vi "mainer.vi"() -> ()   [LabVIEW 2017]
uses:
  mark_10_setting_1.ctl
  acquire_enum.ctl
  serial_setting_1.ctl
  <vilib>/DAQmx/read.llb/DAQmx Read (Analog 1D Wfm NChan NSamp).vi
  <vilib>/DAQmx/miscellaneous.llb/DAQmx Fill In Error Info.vi
  <vilib>/Instr/_visa.llb/VISA Configure Serial Port (Instr).vi
panel:
  in  "Trigger Force(N)":dbl
  in  "Stop Trigger":bool
  in  "Move":bool
  in  "Target Distance":dbl
  in  "Sampling Rate(Hz)":dbl
  out "dt(ms)":u32
  in  "Reset Cycle":bool
  out "Readings":cluster{dbl, "Numeric":dbl, "Numeric":dbl}(graph)
  in  "Record":bool
  in  "Log TXT file":path
  out "Cycles":string
  in  "Zero":bool
  in  "Stop Button":bool
  out "Current Status":string
  in  "Auto Zero":bool
  out "Travel":string
  out "Load":string
  in  "Mark-10":refnum<visa-resource-name>
  in  "Down Button":bool
  in  "Up Button":bool
  in  "Exit":bool
  in  "Mark-10 Setup":bool
  # "Max 45Hz!"
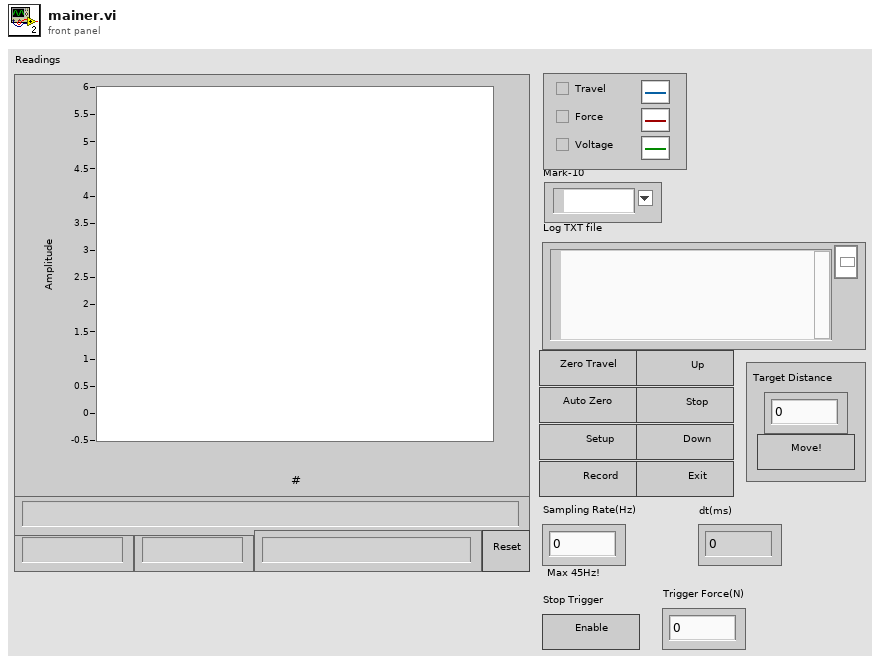
[diagram p1: front panel]
types:
  T1 = typedef "acquire_enum.ctl" = enum16{"Move to Target", "Connect to NIDAQ", "Connect to Mark-10", "Reset Cycle", "Open Mark-10 Setup", "Auto Zero", "Zero", "Stop", "Down", "Up", "Initialize", "Exit", "New Log Path", "Acquire"}
  T2 = typedef "mark_10_setting_1.ctl" = cluster{"Speed (mm/min)":dbl, "Up Limit(mm)":dbl, "Down Limit(mm)":dbl, "Cycle Mode":bool, "Number of Cycles":i32, "IsConfigured":bool}
  T3 = cluster{"Move":refnum<vi>, "Mark-10":refnum<vi>, "Mark-10 Setup":refnum<vi>, "Reset Cycle":refnum<vi>, "Stop Button":refnum<vi>, "Log TXT file":refnum<vi>, "Up Button":refnum<vi>, "Down Button":refnum<vi>, "Auto Zero":refnum<vi>, "Zero":refnum<vi>, "Exit":refnum<vi>, "Record":refnum<vi>, "Sampling Rate(Hz)":refnum<vi>}
  T4 = enum8{"Enabled", "Disabled", "Disabled and Grayed Out"}
  T5 = typedef "serial_setting_1.ctl" = cluster{"baud rate":u32, "data bits":u16, "parity":enum16{"None", "Odd", "Even", "Mark", "Space"}, "stop bits":u16, "flow control":u16, "IsConfigured":bool}
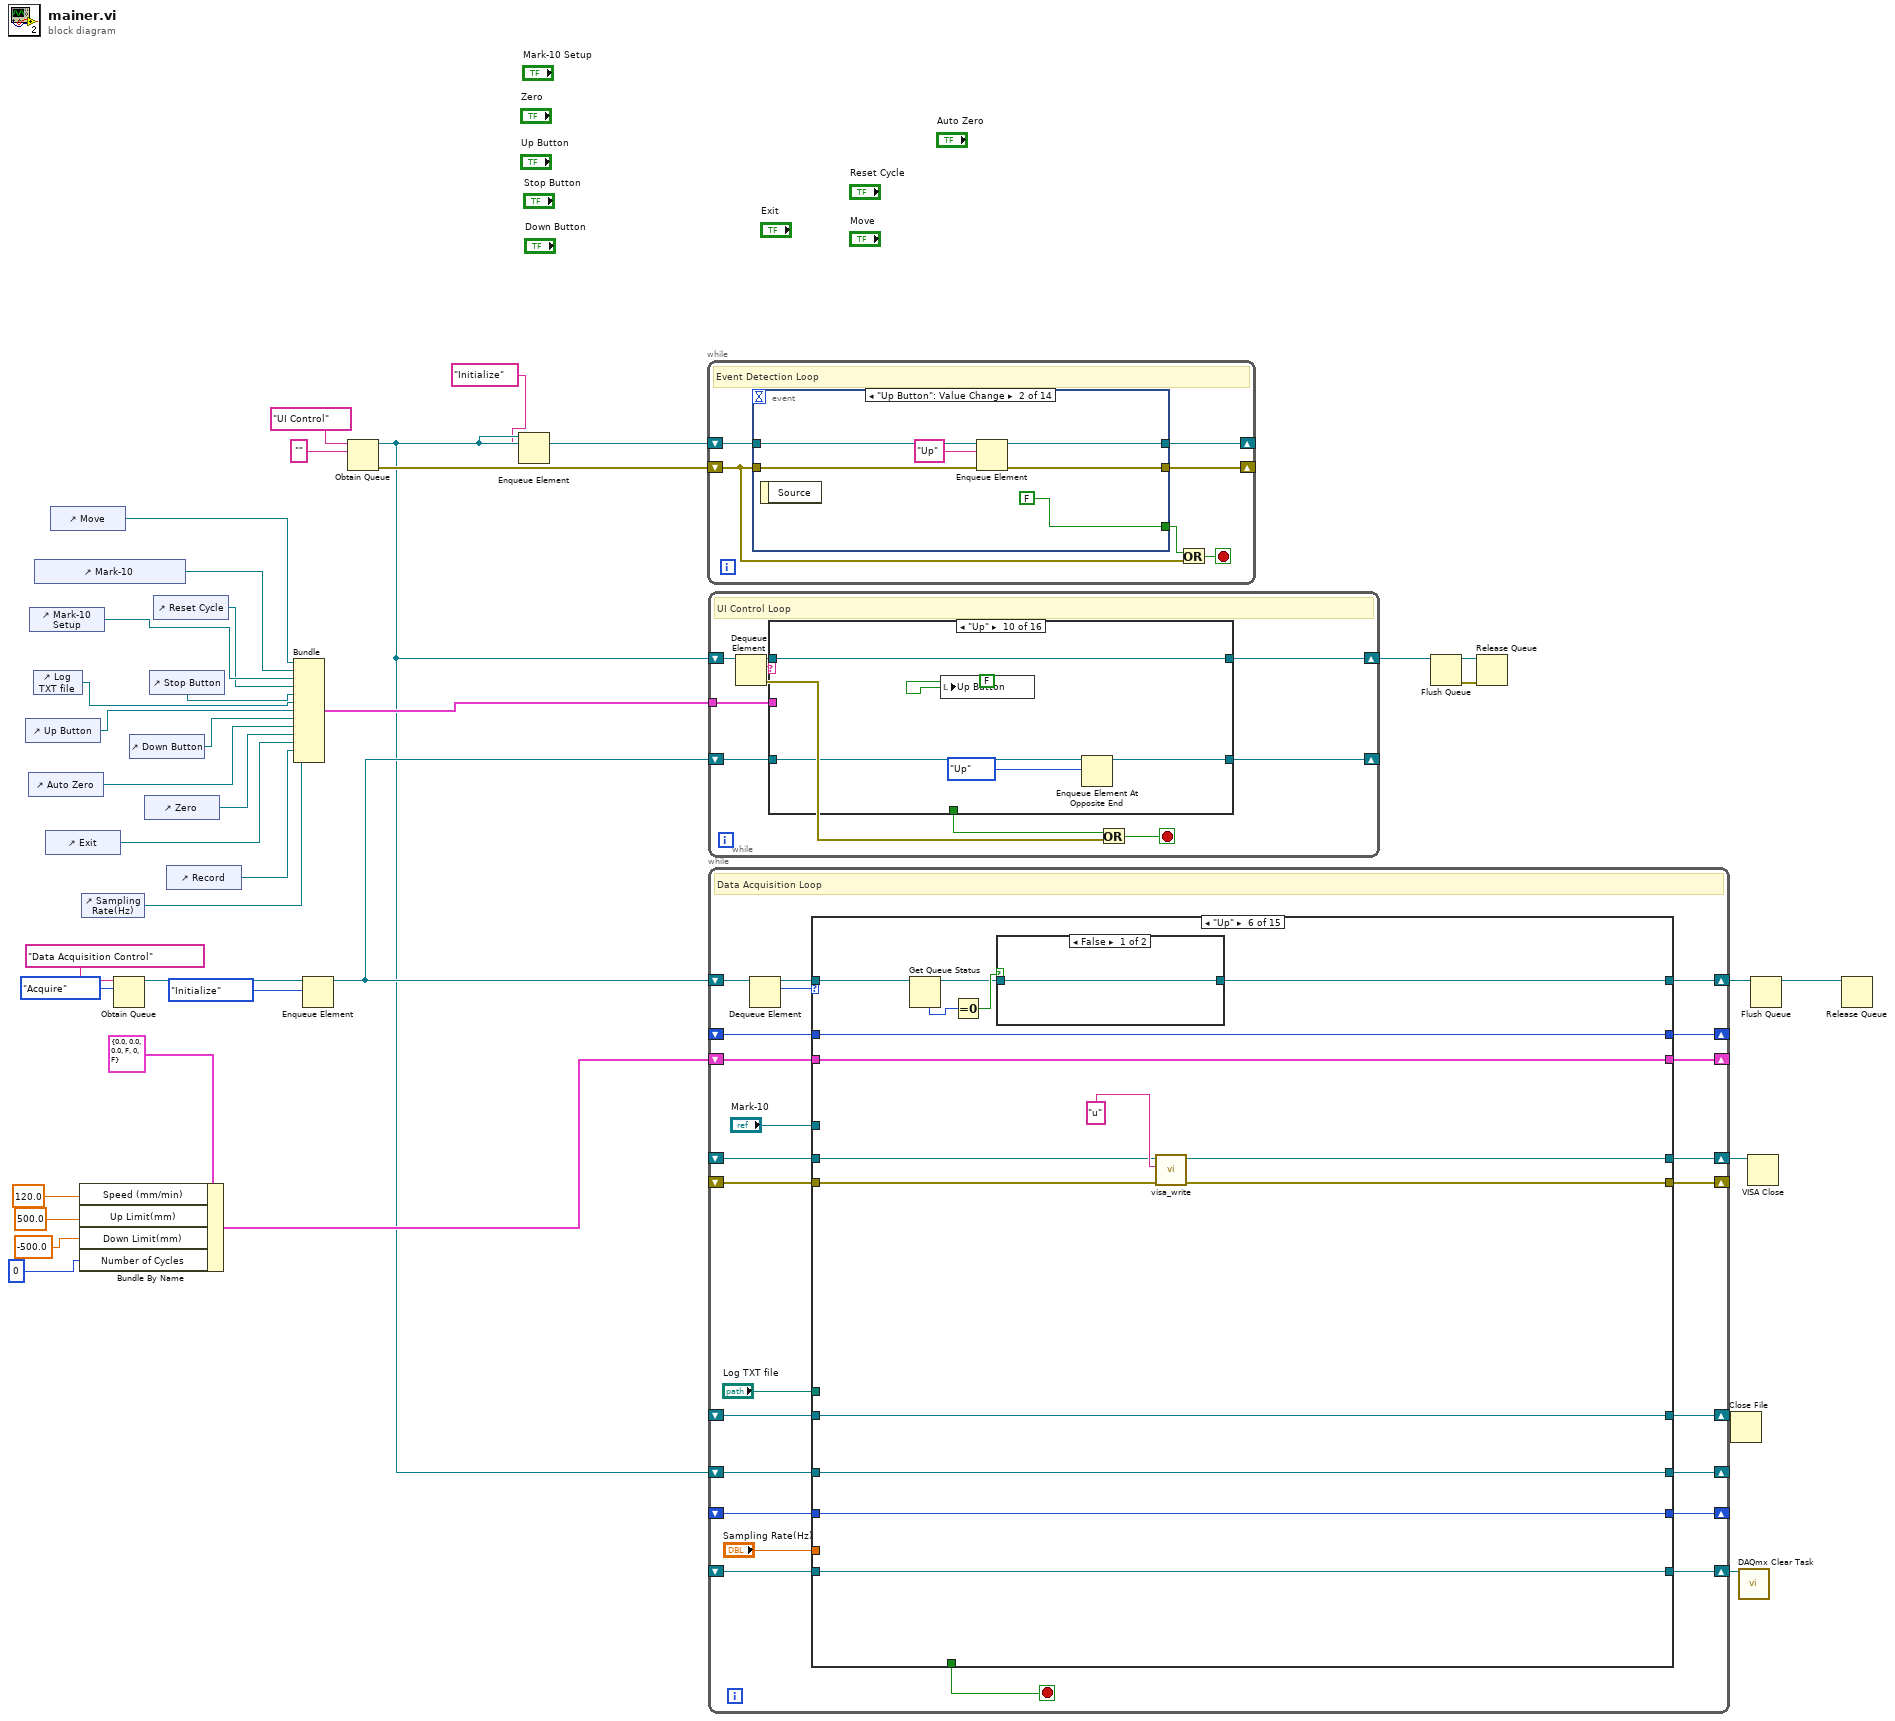
[diagram p0: block diagram]
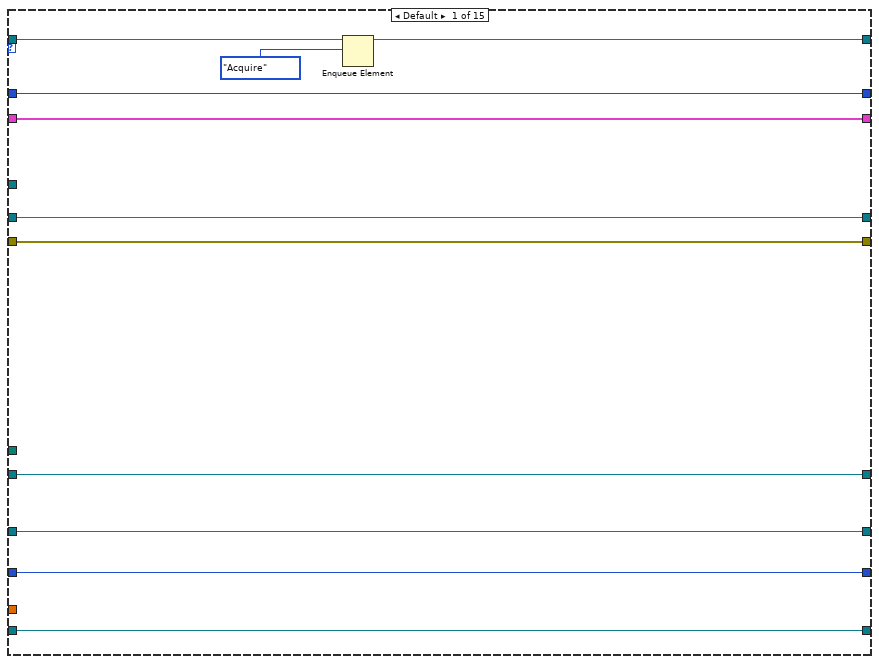
[diagram p2: hidden frame]
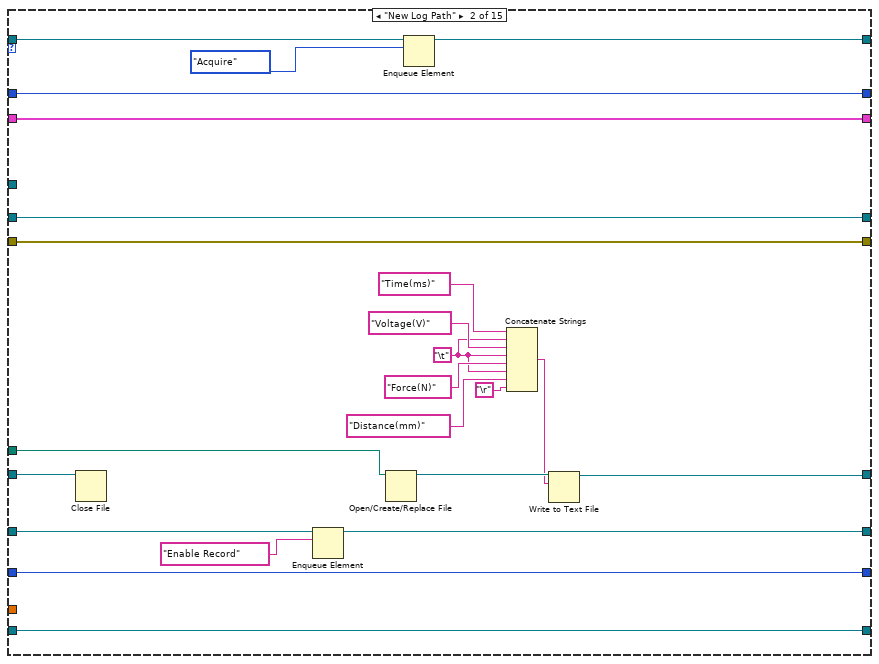
[diagram p3: hidden frame]
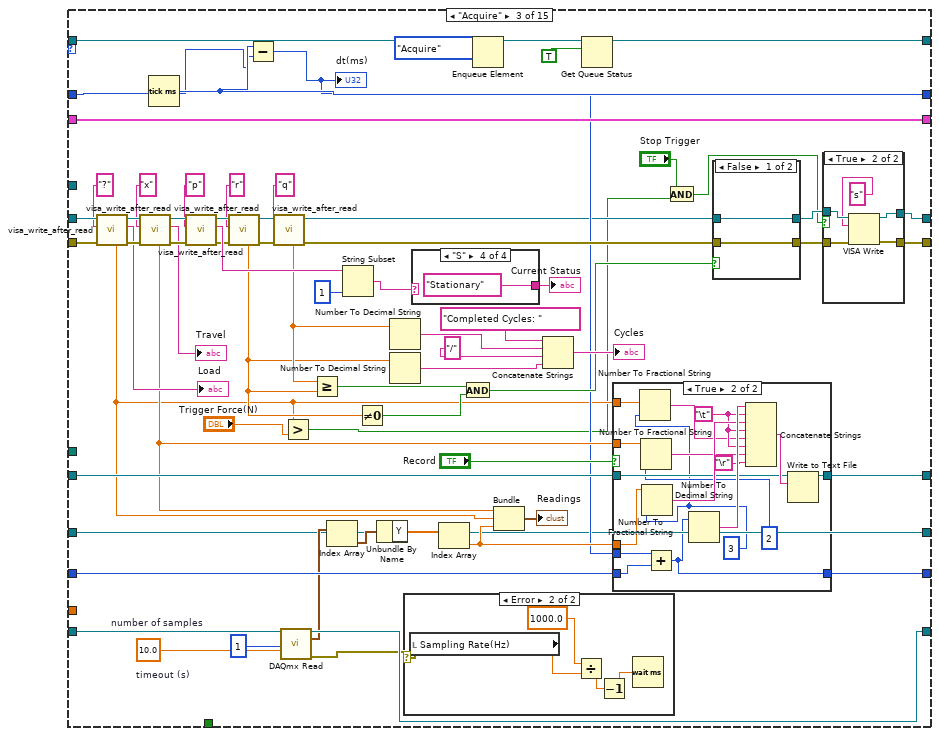
[diagram p4: hidden frame]
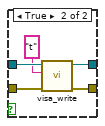
[diagram p7: hidden frame]
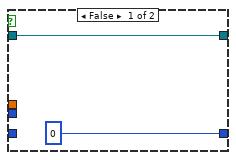
[diagram p8: hidden frame]
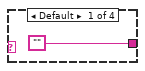
[diagram p9: hidden frame]
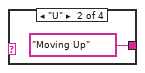
[diagram p10: hidden frame]
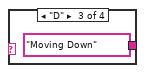
[diagram p11: hidden frame]
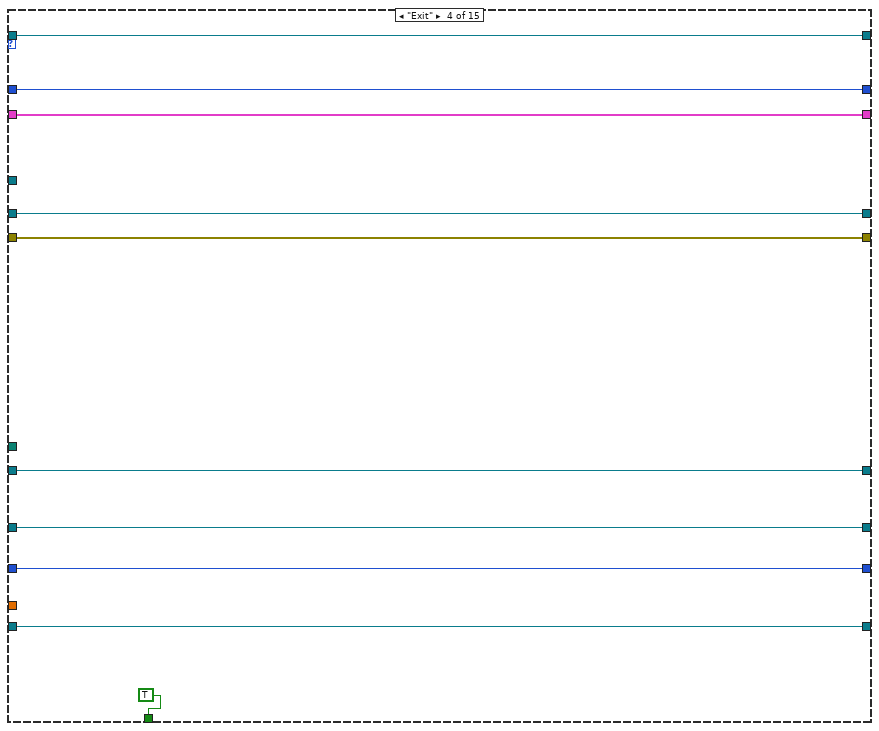
[diagram p12: hidden frame]
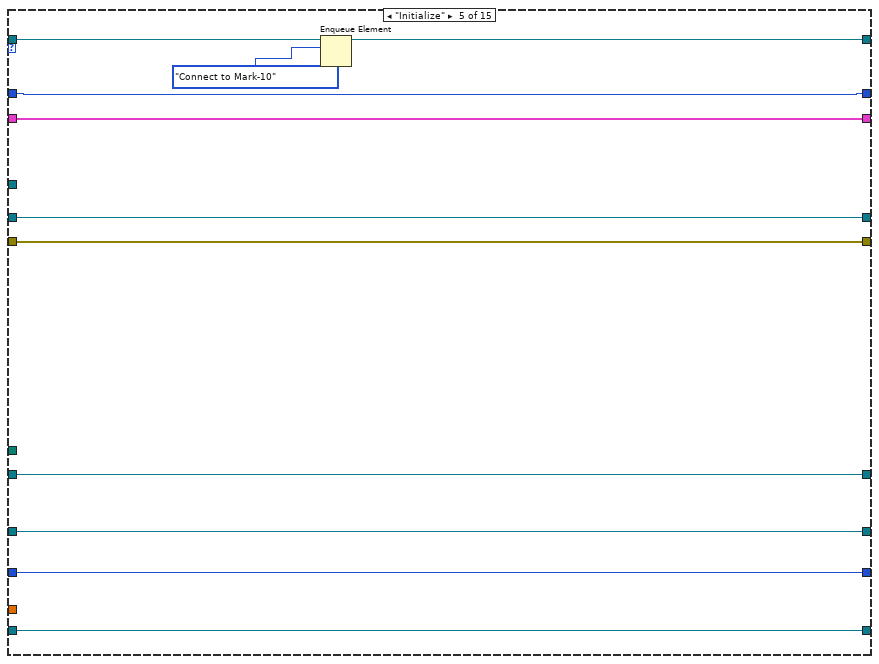
[diagram p13: hidden frame]
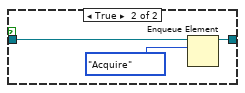
[diagram p14: hidden frame]
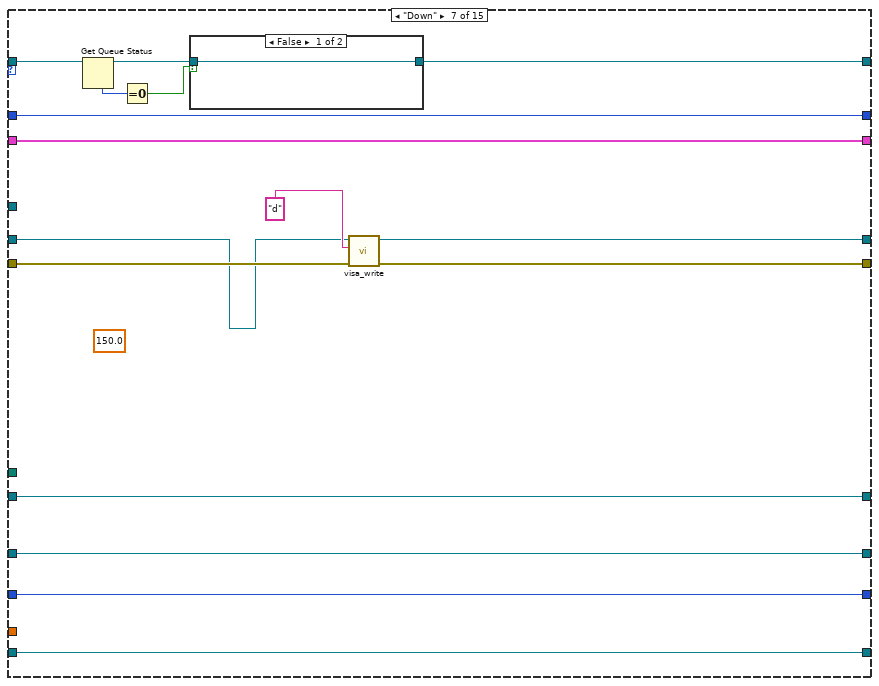
[diagram p15: hidden frame]
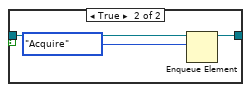
[diagram p16: hidden frame]
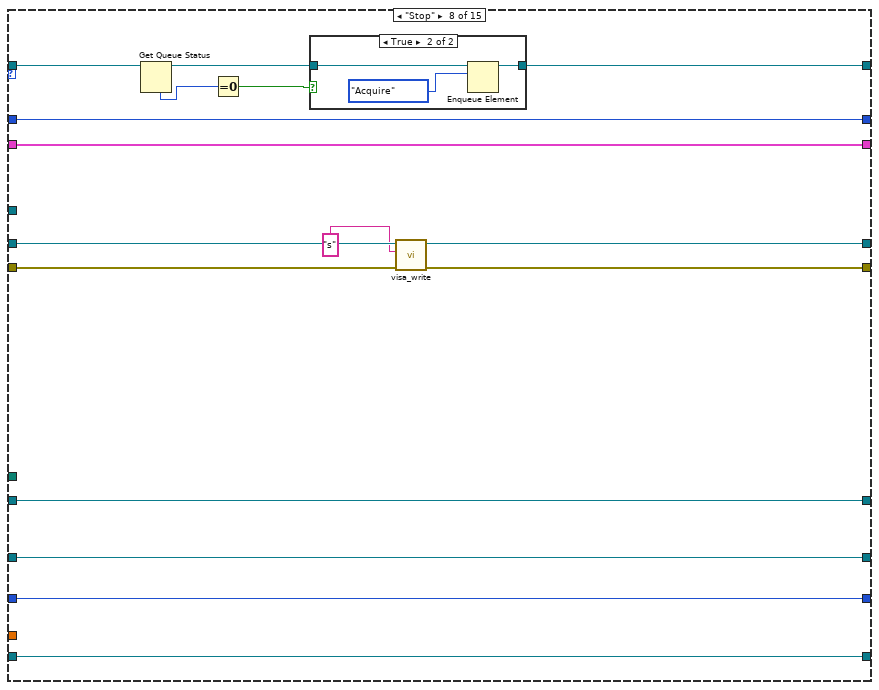
[diagram p17: hidden frame]
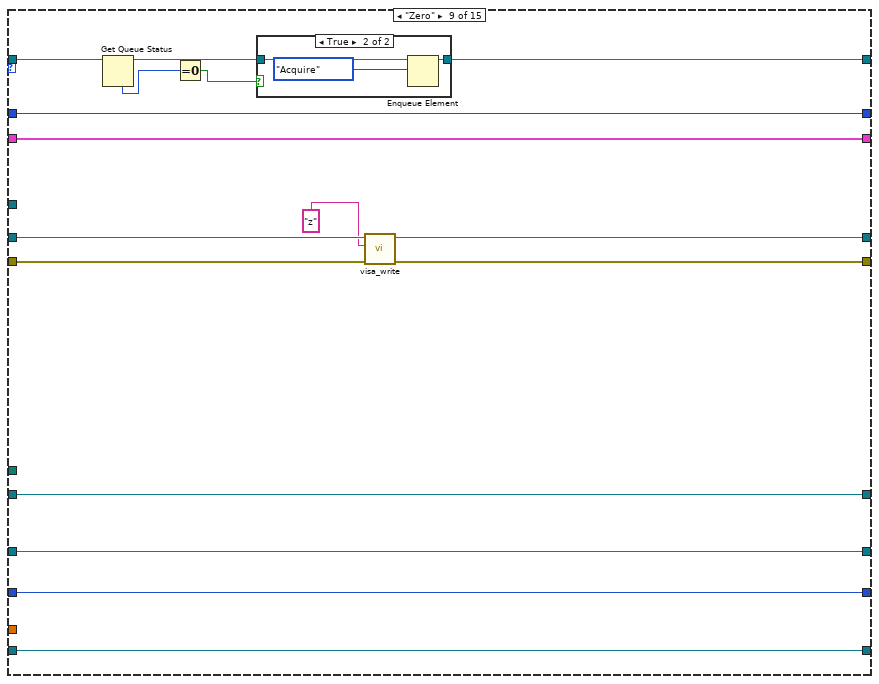
[diagram p19: hidden frame]
diagram:
  n1 = control-ref of="Up Button"() -> (w9:refnum<vi>)
  n2 = control-ref of="Auto Zero"() -> (w7:refnum<vi>)
  n3 = control-ref of="Mark-10 Setup"() -> (w13:refnum<vi>)
  n4 = control-ref of="Log TXT file"() -> (w10:refnum<vi>)
  n5 = control-ref of="Mark-10"() -> (w14:refnum<vi>)
  n6 = control-ref of="Exit"() -> (w5:refnum<vi>)
  n7 = control-ref of="Move"() -> (w15:refnum<vi>)
  n8 = Bundle By Name(cluster=T2 {"Speed (mm/min)"=0.0, "Up Limit(mm)"=0.0, "Down Limit(mm)"=0.0, "Cycle Mode"=FALSE, "Number of Cycles"=0, "IsConfigured"=FALSE} ("Mark-10 Settings"), "Speed (mm/min)"=120.0, "Up Limit(mm)"=500.0, "Down Limit(mm)"=-500.0, "Number of Cycles"=0) -> (w18:T2)
  n9 = control-ref of="Sampling Rate(Hz)"() -> (w1:refnum<vi>)
  n10 = Obtain Queue(name (unnamed)="Data Acquisition Control", element data type=acquire_enum."Acquire") -> (queue out=w29:refnum<queue>)  [unwired: 3 in, 2 out]
  n11 = control-ref of="Down Button"() -> (w8:refnum<vi>)
  n12 = control-ref of="Zero"() -> (w6:refnum<vi>)
  n13 = control-ref of="Stop Button"() -> (w11:refnum<vi>)
  n14 = control-ref of="Reset Cycle"() -> (w12:refnum<vi>)
  n15 = control-ref of="Record"() -> (w4:refnum<vi>)
  n16 = Bundle("Move"=w15, "Mark-10"=w14, "Mark-10 Setup"=w13, "Reset Cycle"=w12, "Stop Button"=w11, "Log TXT file"=w10, "Up Button"=w9, "Down Button"=w8, "Auto Zero"=w7, "Zero"=w6, "Exit"=w5, "Record"=w4, "Sampling Rate(Hz)"=w1) -> (w16:T3)  [unwired: 1 in]
  n17 = Enqueue Element(queue=w29, element=acquire_enum."Initialize") -> (queue out=w27:refnum<queue>)  [unwired: 2 in, 2 out]
  n18 = Obtain Queue(name (unnamed)="UI Control", element data type="") -> (queue out=w3:refnum<queue>, error out=w35:errorcluster)  [unwired: 3 in, 1 out]
  n19 = Enqueue Element(queue=w3, element="Initialize") -> ()  [unwired: 2 in, 3 out]
  n20 = while {
    shift-right: [w43] -> _
    shift-left: w3 -> [w44]
    shift-right: [w42] -> _
    shift-left: w35 -> [w39]
    stop <- w41 stop-if-true
    # "Event Detection Loop"
    n21 = event shown="[1] \"Up Button\": Value Change" {
      selector: _ -> [_ _ _ _ _ _ _ _ _ _ _ _ _ _]
      dyn-events: _ -> [_ _ _ _ _ _ _ _ _ _ _ _ _ _]
      timeout: _ -> [_ _ _ _ _ _ _ _ _ _ _ _ _ _]
      tunnel: [TRUE FALSE FALSE FALSE _ FALSE FALSE FALSE FALSE FALSE FALSE FALSE FALSE TRUE] -> w40
      tunnel: w44 -> [w47 w53 w59 w65 w70 w76 w82 w88 w94 w99 w105 w111 w117 w120]
      tunnel: [w47 w52 w58 w64 w69 w75 w81 w87 w93 w98 w104 w110 w116 w123] -> w43
      tunnel: w39 -> [w46 w51 w57 w63 w67 w74 w80 w86 w92 w97 w103 w109 w115 w119]
      tunnel: [w46 w50 w56 w62 w68 w73 w79 w85 w91 w96 w102 w108 w114 w122] -> w42
      event Timeout {
        n22 = event-data() -> ()  [unwired: 1 in, 1 out]
      }
      event "Up Button": Value Change {
        n23 = event-data() -> ()  [unwired: 1 in, 1 out]
        n24 = Enqueue Element(queue=w53, element="Up", error in (no error)=w51) -> (queue out=w52:refnum<queue>, error out=w50:errorcluster)  [unwired: 1 in, 1 out]
      }
      event "Reset Cycle": Value Change {
        n25 = event-data() -> ()  [unwired: 1 in, 1 out]
        n26 = Enqueue Element(queue=w59, element="Reset Cycle", error in (no error)=w57) -> (queue out=w58:refnum<queue>, error out=w56:errorcluster)  [unwired: 1 in, 1 out]
      }
      event "Stop Button": Value Change {
        n27 = event-data() -> ()  [unwired: 1 in, 2 out]
        n28 = Enqueue Element(queue=w65, element="Stop", error in (no error)=w63) -> (queue out=w64:refnum<queue>, error out=w62:errorcluster)  [unwired: 1 in, 1 out]
      }
      event "Record": Value Change {
        n29 = event-data() -> ()  [unwired: 1 in, 2 out]
        n30 = Enqueue Element(queue=w70, element="Record", error in (no error)=w67) -> (queue out=w69:refnum<queue>, error out=w68:errorcluster)  [unwired: 1 in, 1 out]
      }
      event "Log TXT file": Value Change {
        n31 = event-data() -> ()  [unwired: 1 in, 2 out]
        n32 = Enqueue Element(queue=w76, element="Change Log Path", error in (no error)=w74) -> (queue out=w75:refnum<queue>, error out=w73:errorcluster)  [unwired: 1 in, 1 out]
      }
      event "Sampling Rate(Hz)": Value Change {
        n33 = event-data() -> ()  [unwired: 1 in, 2 out]
        n34 = Enqueue Element(queue=w82, element="Change Sampling Rate", error in (no error)=w80) -> (queue out=w81:refnum<queue>, error out=w79:errorcluster)  [unwired: 1 in, 1 out]
      }
      event "Move": Value Change {
        n35 = event-data() -> ()  [unwired: 1 in, 2 out]
        n36 = Enqueue Element(queue=w88, element="Move", error in (no error)=w86) -> (queue out=w87:refnum<queue>, error out=w85:errorcluster)  [unwired: 1 in, 1 out]
      }
      event "Zero": Value Change {
        n37 = event-data() -> ()  [unwired: 1 in, 2 out]
        n38 = Enqueue Element(queue=w94, element="Zero", error in (no error)=w92) -> (queue out=w93:refnum<queue>, error out=w91:errorcluster)  [unwired: 1 in, 1 out]
      }
      event "Down Button": Value Change {
        n39 = event-data() -> ()  [unwired: 1 in, 1 out]
        n40 = Enqueue Element(queue=w99, element="Down", error in (no error)=w97) -> (queue out=w98:refnum<queue>, error out=w96:errorcluster)  [unwired: 1 in, 1 out]
      }
      event "Mark-10": Value Change {
        n41 = event-data() -> ()  [unwired: 1 in, 2 out]
        n42 = Enqueue Element(queue=w105, element="Connect to Mark-10", error in (no error)=w103) -> (queue out=w104:refnum<queue>, error out=w102:errorcluster)  [unwired: 1 in, 1 out]
      }
      event "Mark-10 Setup": Value Change {
        n43 = event-data() -> ()  [unwired: 1 in, 2 out]
        n44 = Enqueue Element(queue=w111, element="Open Mark-10 Setup", error in (no error)=w109) -> (queue out=w110:refnum<queue>, error out=w108:errorcluster)  [unwired: 1 in, 1 out]
      }
      event "Auto Zero": Value Change {
        n45 = event-data() -> ()  [unwired: 1 in, 2 out]
        n46 = Enqueue Element(queue=w117, element="Auto Zero", error in (no error)=w115) -> (queue out=w116:refnum<queue>, error out=w114:errorcluster)  [unwired: 1 in, 1 out]
      }
      event "Exit": Value Change {
        n47 = event-data() -> ()  [unwired: 1 in, 1 out]
        n48 = Enqueue Element(queue=w120, element="Exit", error in (no error)=w119) -> (queue out=w123:refnum<queue>, error out=w122:errorcluster)  [unwired: 1 in, 1 out]
      }
    }
    n49 = Or(x=w40, y=w39) -> (x .or. y?=w41:bool)
  }
  n50 = while {
    shift-right: [w131] -> w25
    shift-left: w3 -> [w134]
    shift-right: [w129] -> _
    shift-left: w27 -> [w130]
    tunnel: w16 -> [w125]
    stop <- w128 stop-if-true
    # "UI Control Loop"
    n51 = Dequeue Element(queue=w134) -> (queue out=w132:refnum<queue>, element=w133:string, error out=w126:errorcluster)  [unwired: 2 in, 1 out]
    n52 = case shown="\"Up\"" w133 {
      tunnel: w132 -> [w136 w137 w145 w150 w154 w159 w163 w167 w172 w173 w179 w189 w194 w199 w204 w209]
      tunnel: [w136 w137 w145 w150 w154 w159 w163 w167 w172 w173 w179 w189 w194 w199 w204 w209] -> w131
      tunnel: [_ _ TRUE _ _ _ _ _ _ _ _ _ _ _ _ _] -> w127
      tunnel: w130 -> [w135 w138 w143 w147 w153 w158 w162 w166 w171 w175 w178 w188 w191 w196 w202 w207]
      tunnel: [w135 w138 w142 w146 w152 w156 w160 w164 w169 w174 w178 w188 w190 w195 w201 w206] -> w129
      tunnel: w125 -> [_ _ _ _ _ _ _ _ _ _ _ w187 _ _ _ _]
      frame Default {
      }
      frame "Record" {
        n53 = control-ref of="Log TXT file"() -> (w139:refnum<vi>)
        n54 = call "toggle_enable.vi"("reference"=w139) -> ()  [unwired: 10 in, 1 out]
      }
      frame "Exit" {
        n55 = local write "Exit"(FALSE) -> ()
        n56 = Enqueue Element(queue=w143, element=acquire_enum."Exit") -> (queue out=w142:refnum<queue>)  [unwired: 2 in, 2 out]
      }
      frame "Open Mark-10 Setup" {
        n57 = local write "Mark-10 Setup"(FALSE) -> ()
        n58 = Enqueue Element(queue=w147, element=acquire_enum."Open Mark-10 Setup") -> (queue out=w146:refnum<queue>)  [unwired: 2 in, 2 out]
      }
      frame "Auto Zero" {
        n59 = local write "Auto Zero"(FALSE) -> ()
        n60 = Enqueue Element(queue=w153, element=acquire_enum."Auto Zero") -> (queue out=w152:refnum<queue>)  [unwired: 2 in, 2 out]
      }
      frame "Change Log Path" {
        n61 = Enqueue Element(queue=w158, element=acquire_enum."New Log Path") -> (queue out=w156:refnum<queue>)  [unwired: 2 in, 2 out]
      }
      frame "Connect to Mark-10" {
        n62 = Enqueue Element(queue=w162, element=acquire_enum."Connect to Mark-10") -> (queue out=w160:refnum<queue>)  [unwired: 2 in, 2 out]
      }
      frame "Change Sampling Rate" {
        n63 = Enqueue Element(queue=w166, element=acquire_enum."Connect to NIDAQ") -> (queue out=w164:refnum<queue>)  [unwired: 2 in, 2 out]
      }
      frame "Move" {
        n64 = Enqueue Element(queue=w171, element=acquire_enum."Move to Target") -> (queue out=w169:refnum<queue>)  [unwired: 2 in, 2 out]
        n65 = local write "Move"(FALSE) -> ()
      }
      frame "Up" {
        n66 = local write "Up Button"(FALSE) -> ()
        n67 = Enqueue Element At Opposite End(queue=w175, element=acquire_enum."Up") -> (queue out=w174:refnum<queue>)  [unwired: 2 in, 2 out]
      }
      frame "Enable Record" {
        n68 = local write "Record"(FALSE) -> ()
        n69 = property on="Log TXT file" class="Path"("DisabledEnum"=T4."Enabled" ("Disabled")) -> ()  [unwired: 2 in, 2 out]
      }
      frame "Initialize" {
        n70 = Unbundle By Name(w187) -> ("Up Button"=w184:refnum<vi>, "Down Button"=w186:refnum<vi>, "Record"=w185:refnum<vi>)
        n71 = Build Array(w184, w186, w185) -> (w183:refnum<vi>[])
        n72 = call "disable_and_gray_out_buttons.vi"("Disabled"=T4."Enabled", "Array"=w183) -> ()  [unwired: 10 in]
      }
      frame "Reset Cycle" {
        n73 = local write "Reset Cycle"(FALSE) -> ()
        n74 = Enqueue Element(queue=w191, element=acquire_enum."Reset Cycle") -> (queue out=w190:refnum<queue>)  [unwired: 2 in, 2 out]
      }
      frame "Stop" {
        n75 = local write "Stop Button"(FALSE) -> ()
        n76 = Enqueue Element At Opposite End(queue=w196, element=acquire_enum."Stop") -> (queue out=w195:refnum<queue>)  [unwired: 2 in, 2 out]
      }
      frame "Zero" {
        n77 = local write "Zero"(FALSE) -> ()
        n78 = Enqueue Element At Opposite End(queue=w202, element=acquire_enum."Zero") -> (queue out=w201:refnum<queue>)  [unwired: 2 in, 2 out]
      }
      frame "Down" {
        n79 = local write "Down Button"(FALSE) -> ()
        n80 = Enqueue Element At Opposite End(queue=w207, element=acquire_enum."Down") -> (queue out=w206:refnum<queue>)  [unwired: 2 in, 2 out]
      }
    }
    n81 = Or(x=w127, y=w126) -> (x .or. y?=w128:bool)
  }
  n82 = while {
    shift-right: [w214] -> w26
    shift-left: _ -> [w233]
    shift-right: [w217] -> _
    shift-left: _ -> [w220]
    shift-right: [w231] -> w33
    shift-left: _ -> [w232]
    shift-right: [w229] -> w32
    shift-left: _ -> [w230]
    shift-right: [w228] -> _
    shift-left: _ -> [w227]
    shift-right: [w226] -> _
    shift-left: _ -> [w225]
    shift-right: [w221] -> w24
    shift-left: w27 -> [w223]
    shift-right: [w218] -> _
    shift-left: w18 -> [w219]
    shift-right: [w211] -> _
    shift-left: w3 -> [w212]
    stop <- w216 stop-if-true
    # "Data Acquisition Loop"
    n83 = Dequeue Element(queue=w223) -> (queue out=w222:refnum<queue>, element=w224:T1)  [unwired: 2 in, 2 out]
    n84 = case shown="\"Up\"" w224 {
      tunnel: w233 -> [w243 w265 w335 w384 w393 w398 w418 w451 w471 w490 w547 w572 _ w626 w668]
      tunnel: w220 -> [w242 w264 w334 w383 w392 w413 w433 w448 w468 w489 w546 w571 _ w627 w660]
      tunnel: w232 -> [w239 w262 w333 w380 w389 w407 w426 w445 w464 w516 w539 w564 w595 w619 w661]
      tunnel: [w239 w262 w332 w380 w389 w407 w426 w445 w464 w516 w539 w564 w595 w629 w661] -> w231
      tunnel: w230 -> [w241 w267 w331 w382 w391 w409 w428 w447 w466 w518 w541 w566 w597 w628 w663]
      tunnel: [w241 w250 w330 w382 w391 w409 w428 w447 w466 w518 w541 w566 w597 w628 w663] -> w229
      tunnel: [w240 w263 w329 w381 w390 w408 w427 w446 w465 w517 w540 w565 w596 w620 w662] -> w228
      tunnel: w227 -> [w240 w263 w328 w381 w390 w408 w427 w446 w465 w517 w540 w565 w596 w620 w662]
      tunnel: [w244 w266 w301 w385 w394 w406 w429 w452 w472 w519 w538 w567 w598 w624 w664] -> w226
      tunnel: w225 -> [w244 w266 w300 w385 w394 w406 w429 w452 w472 w519 w538 w567 w598 w624 w664]
      tunnel: w222 -> [w237 w260 w283 w386 w397 w402 w422 w442 w461 w496 w555 w574 w600 w622 w655]
      tunnel: [w236 w259 w284 w386 w395 w405 w430 w453 w473 w492 w556 w575 w599 w621 w651] -> w221
      tunnel: [_ _ _ TRUE _ _ _ _ _ _ _ _ _ _ _] -> w216
      tunnel: w219 -> [w235 w258 w281 w378 w388 w400 w420 w439 w459 w491 w545 w568 w589 w625 w656]
      tunnel: [w235 w258 w281 w378 w388 w400 w420 w439 w459 w483 w544 w568 w589 w625 w656] -> w218
      tunnel: [w242 w264 w275 w383 w392 w412 w431 w449 w469 w479 w542 w569 w584 w627 w641] -> w217
      tunnel: "Mark-10" -> [_ _ _ _ _ _ _ _ _ _ _ _ w594 _ _]
      tunnel: [w243 w265 w273 w384 w393 w411 w432 w450 w470 w482 w543 w570 w586 w626 w643] -> w214
      tunnel: "Log TXT file" -> [_ w248 _ _ _ _ _ _ _ _ _ _ _ _ _]
      tunnel: [w234 w246 w278 w377 w387 w399 w419 w438 w458 w478 w535 w563 w585 w618 w631] -> w211
      tunnel: w212 -> [w234 w247 w278 w377 w387 w399 w419 w438 w458 w478 w535 w563 w585 w618 w631]
      tunnel: "Sampling Rate(Hz)" -> [_ _ _ _ _ _ _ _ _ _ _ _ _ w617 _]
      frame Default {
        n85 = Enqueue Element(queue=w237, element=acquire_enum."Acquire") -> (queue out=w236:refnum<queue>)  [unwired: 2 in, 2 out]
      }
      frame "New Log Path" {
        w254 = "\t"
        n86 = Close File(refnum=w267) -> ()  [unwired: 1 in, 2 out]
        n87 = Enqueue Element(queue=w247, element="Enable Record") -> (queue out=w246:refnum<queue>)  [unwired: 2 in, 2 out]
        n88 = Open/Create/Replace File(file path (use dialog)=w248) -> (refnum out=w251:refnum<file>)  [unwired: 5 in, 2 out]
        n89 = Enqueue Element(queue=w260, element=acquire_enum."Acquire") -> (queue out=w259:refnum<queue>)  [unwired: 2 in, 2 out]
        n90 = Concatenate Strings("Time(ms)", w254, "Voltage(V)", w254, "Force(N)", w254, "Distance(mm)", "\r") -> (w249:string)
        n91 = Write to Text File(file (use dialog)=w251, text=w249) -> (refnum out=w250:refnum<file>)  [unwired: 2 in, 2 out]
      }
      frame "Acquire" {
        w303 = 1  # number of samples
        w318 = 10.0  # timeout (s)
        n92 = call "visa_write_after_read.vi"("error in (no error)"=w334, "String"="?", "VISA Refnum in"=w335) -> ("error out"=w324:errorcluster, "trimmed string"=→"Load":string, "VISA Refnum out"=w323:refnum<visa-resource-name>, "Numeric"=w269:dbl)  [unwired: 5 in]
        n93 = call "visa_write_after_read.vi"("error in (no error)"=w324, "String"="x", "VISA Refnum in"=w323) -> ("error out"=w320:errorcluster, "trimmed string"=→"Travel":string, "VISA Refnum out"=w321:refnum<visa-resource-name>, "Numeric"=w302:dbl)  [unwired: 5 in]
        n94 = Tick Count (ms)() -> (millisecond timer value=w301:u32)
        n95 = call "visa_write_after_read.vi"("error in (no error)"=w320, "String"="p", "VISA Refnum in"=w321) -> ("error out"=w296:errorcluster, "trimmed string"=w319:string, "VISA Refnum out"=w298:refnum<visa-resource-name>)  [unwired: 5 in, 1 out]
        n96 = call "visa_write_after_read.vi"("error in (no error)"=w296, "String"="r", "VISA Refnum in"=w298) -> ("error out"=w295:errorcluster, "VISA Refnum out"=w297:refnum<visa-resource-name>, "Numeric"=w289:dbl)  [unwired: 5 in, 1 out]
        n97 = Subtract(x=w301, y=w300) -> (x-y=w280:u32)
        "dt(ms)" <- w280
        n98 = call "visa_write_after_read.vi"("error in (no error)"=w295, "String"="q", "VISA Refnum in"=w297) -> ("error out"=w291:errorcluster, "VISA Refnum out"=w277:refnum<visa-resource-name>, "Numeric"=w290:dbl)  [unwired: 5 in, 1 out]
        n99 = call-poly <vilib>:"DAQmx Read.vi"("task/channels in"=w333, "number of samples per channel"=w303, "timeout"=w318) -> ("task out"=w332:refnum<k21>, "data"=w317:waveform(dbl)[], "error out"=w279:errorcluster)  [unwired: 10 in]
        n100 = Greater?(x=w269, y="Trigger Force(N)") -> (0:w268:bool)
        n101 = Greater Or Equal?(x=w290, y=w289) -> (x >= y?=w288:bool)
        n102 = Index Array(array=w317) -> (element=w316:waveform(dbl))  [unwired: 1 in]
        n103 = String Subset(string=w319, length (rest)=1) -> (substring=w325:string)  [unwired: 1 in]
        n104 = Not Equal To 0?(x=w289) -> (x != 0?=w287:bool)
        n105 = Unbundle By Name(w316) -> ("Y"=w306:dbl[])
        n106 = Number To Decimal String(number=w290) -> (decimal integer string=w307:string)  [unwired: 1 in]
        n107 = Number To Decimal String(number=w289) -> (decimal integer string=w308:string)  [unwired: 1 in]
        n108 = case shown="Error" w279 {
          frame No Error {
          }
          frame Error {
            n109 = local read "Sampling Rate(Hz)"() -> (w346:dbl)
            n110 = Divide(x=1000.0, y=w346) -> (x/y=w343:dbl)
            n111 = Decrement(x=w343) -> (x-1=w344:dbl)
            n112 = Wait (ms)(milliseconds to wait=w344) -> ()  [unwired: 1 out]
          }
        }
        n113 = case shown="\"S\"" w325 {
          tunnel: ["" "Moving Up" "Moving Down" "Stationary"] -> w309
          frame Default {
          }
          frame "U" {
          }
          frame "D" {
          }
          frame "S" {
          }
        }
        "Current Status" <- w309
        n114 = Index Array(array=w306) -> (element=w304:dbl)  [unwired: 1 in]
        n115 = And(x=w288, y=w287) -> (x .and. y?=w292:bool)
        n116 = Enqueue Element(queue=w283, element=acquire_enum."Acquire") -> (queue out=w285:refnum<queue>)  [unwired: 2 in, 2 out]
        n117 = Bundle("Numeric"=w302, "Numeric"=w269, w304) -> (→"Readings":cluster{"Numeric":dbl, "Numeric":dbl, dbl})  [unwired: 1 in]
        n118 = Concatenate Strings("Completed Cycles: ", w307, "/", w308) -> (→"Cycles":string)
        n119 = Get Queue Status(queue=w285, return elements? (F)=TRUE) -> (queue out=w284:refnum<queue>)  [unwired: 1 in, 7 out]
        n120 = case shown="True" "Record" {
          tunnel: w331 -> [w355 w367]
          tunnel: [w355 w366] -> w330
          tunnel: w269 -> [_ w365]
          tunnel: w302 -> [_ w363]
          tunnel: [0 w358] -> w329
          tunnel: w280 -> [_ w360]
          tunnel: w328 -> [_ w359]
          tunnel: w304 -> [_ w361]
          frame False {
          }
          frame True {
            w356 = 3
            w370 = "\t"
            n121 = Number To Fractional String(number=w365, precision (6)=w356) -> (F-format string=w364:string)  [unwired: 2 in]
            n122 = Number To Fractional String(number=w363, precision (6)=2) -> (F-format string=w362:string)  [unwired: 2 in]
            n123 = Number To Fractional String(number=w361, precision (6)=w356) -> (F-format string=w371:string)  [unwired: 2 in]
            n124 = Add(x=w360, y=w359) -> (x+y=w358:u32)
            n125 = Number To Decimal String(number=w358) -> (decimal integer string=w372:string)  [unwired: 1 in]
            n126 = Concatenate Strings(w372, w370, w371, w370, w364, w370, w362, "\r") -> (w368:string)
            n127 = Write to Text File(file (use dialog)=w367, text=w368) -> (refnum out=w366:refnum<file>)  [unwired: 2 in, 2 out]
          }
        }
        n128 = And(x="Stop Trigger", y=w268) -> (x .and. y?=w271:bool)
        n129 = case shown="False" w292 {
          tunnel: w277 -> [w347 w353]
          tunnel: [w347 w351] -> w274
          tunnel: w291 -> [w348 w352]
          tunnel: [w348 w350] -> w276
          frame False {
          }
          frame True {
            n130 = call "visa_write.vi"("error in (no error)"=w352, "String"="t", "VISA Refnum in"=w353) -> ("error out"=w350:errorcluster, "VISA Refnum out"=w351:refnum<visa-resource-name>)  [unwired: 6 in]
          }
        }
        n131 = case shown="True" w271 {
          tunnel: [w337 w342] -> w275
          tunnel: w276 -> [w337 w340]
          tunnel: [w336 w339] -> w273
          tunnel: w274 -> [w336 w341]
          frame False {
          }
          frame True {
            n132 = VISA Write(VISA resource name=w341, write buffer="s", error in (no error)=w340) -> (VISA resource name out=w339:refnum<visa-resource-name>, error out=w342:errorcluster)  [unwired: 1 out]
          }
        }
      }
      frame "Exit" {
      }
      frame "Initialize" {
        n133 = Enqueue Element(queue=w397, element=acquire_enum."Connect to Mark-10") -> (queue out=w395:refnum<queue>)  [unwired: 2 in, 2 out]
      }
      frame "Up" {
        n134 = Get Queue Status(queue=w402) -> (queue out=w401:refnum<queue>, # elements in queue=w404:i32)  [unwired: 2 in, 6 out]
        n135 = Equal To 0?(x=w404) -> (x = 0?=w403:bool)
        n136 = case shown="False" w403 {
          tunnel: w401 -> [w414 w417]
          tunnel: [w414 w416] -> w405
          frame False {
          }
          frame True {
            n137 = Enqueue Element(queue=w417, element=acquire_enum."Acquire") -> (queue out=w416:refnum<queue>)  [unwired: 2 in, 2 out]
          }
        }
        n138 = call "visa_write.vi"("error in (no error)"=w413, "String"="u", "VISA Refnum in"=w398) -> ("error out"=w412:errorcluster, "VISA Refnum out"=w411:refnum<visa-resource-name>)  [unwired: 6 in]
      }
      frame "Down" {
        (unwired) 150.0
        n139 = Get Queue Status(queue=w422) -> (queue out=w421:refnum<queue>, # elements in queue=w424:i32)  [unwired: 2 in, 6 out]
        n140 = Equal To 0?(x=w424) -> (x = 0?=w423:bool)
        n141 = case shown="False" w423 {
          tunnel: w421 -> [w434 w437]
          tunnel: [w434 w436] -> w430
          frame False {
          }
          frame True {
            n142 = Enqueue Element(queue=w437, element=acquire_enum."Acquire") -> (queue out=w436:refnum<queue>)  [unwired: 2 in, 2 out]
          }
        }
        n143 = call "visa_write.vi"("error in (no error)"=w433, "String"="d", "VISA Refnum in"=w418) -> ("error out"=w431:errorcluster, "VISA Refnum out"=w432:refnum<visa-resource-name>)  [unwired: 6 in]
      }
      frame "Stop" {
        n144 = Get Queue Status(queue=w442) -> (queue out=w440:refnum<queue>, # elements in queue=w441:i32)  [unwired: 2 in, 6 out]
        n145 = Equal To 0?(x=w441) -> (x = 0?=w443:bool)
        n146 = case shown="True" w443 {
          tunnel: w440 -> [w454 w457]
          tunnel: [w454 w456] -> w453
          frame False {
          }
          frame True {
            n147 = Enqueue Element(queue=w457, element=acquire_enum."Acquire") -> (queue out=w456:refnum<queue>)  [unwired: 2 in, 2 out]
          }
        }
        n148 = call "visa_write.vi"("error in (no error)"=w448, "String"="s", "VISA Refnum in"=w451) -> ("error out"=w449:errorcluster, "VISA Refnum out"=w450:refnum<visa-resource-name>)  [unwired: 6 in]
      }
      frame "Zero" {
        n149 = Get Queue Status(queue=w461) -> (queue out=w460:refnum<queue>, # elements in queue=w463:i32)  [unwired: 2 in, 6 out]
        n150 = Equal To 0?(x=w463) -> (x = 0?=w462:bool)
        n151 = case shown="True" w462 {
          tunnel: w460 -> [w474 w476]
          tunnel: [w474 w475] -> w473
          frame False {
          }
          frame True {
            n152 = Enqueue Element(queue=w476, element=acquire_enum."Acquire") -> (queue out=w475:refnum<queue>)  [unwired: 2 in, 2 out]
          }
        }
        n153 = call "visa_write.vi"("error in (no error)"=w468, "String"="z", "VISA Refnum in"=w471) -> ("error out"=w469:errorcluster, "VISA Refnum out"=w470:refnum<visa-resource-name>)  [unwired: 6 in]
      }
      frame "Auto Zero" {
        w513 = "\r"
        n154 = Flush Queue(queue=w496) -> (queue out=w495:refnum<queue>)  [unwired: 1 in, 2 out]
        n155 = call "speed_limit_setup.vi"("Down Limit"=-500.0, "Up Limit"=500.0, "Speed"=100.0) -> ("String out"=w512:string, "String out 2"=w511:string, "String out 3"=w510:string)  [unwired: 6 in]
        n156 = Concatenate Strings(w510, w513, w511, w513, w512, w513, "d") -> (w515:string)
        n157 = VISA Write(VISA resource name=w490, write buffer=w515, error in (no error)=w489) -> (VISA resource name out=w500:refnum<visa-resource-name>, error out=w501:errorcluster)  [unwired: 1 out]
        n158 = while {
          shift-right: [w527] -> w502
          shift-left: w500 -> [w529]
          shift-right: [w525] -> w503
          shift-left: w501 -> [w528]
          shift-right: [w523] -> w493
          shift-left: w495 -> [w524]
          shift-right: [w533] -> w483
          shift-left: w491 -> [w533]
          stop <- w531 stop-if-true
          n159 = Get Queue Status(queue=w524) -> (queue out=w523:refnum<queue>, # elements in queue=w521:i32)  [unwired: 2 in, 6 out]
          n160 = call "visa_write_after_read.vi"("error in (no error)"=w528, "String"="?", "VISA Refnum in"=w529) -> ("error out"=w525:errorcluster, "VISA Refnum out"=w527:refnum<visa-resource-name>, "Numeric"=w526:dbl)  [unwired: 5 in, 1 out]
          n161 = Greater Or Equal?(x=w526, y=4.0) -> (x >= y?=w532:bool)
          n162 = Not Equal?(x=w521, y=0) -> (x != y?=w520:bool)
          n163 = Or(x=w520, y=w532) -> (x .or. y?=w531:bool)
        }
        n164 = Concatenate Strings("s", "\r", "z") -> (w507:string)
        n165 = Unbundle By Name(w483) -> ("Speed (mm/min)"=w487:dbl, "Up Limit(mm)"=w484:dbl, "Down Limit(mm)"=w485:dbl, "Number of Cycles"=w486:i32)
        n166 = VISA Write(VISA resource name=w502, write buffer=w507, error in (no error)=w503) -> (VISA resource name out=w508:refnum<visa-resource-name>, error out=w509:errorcluster)  [unwired: 1 out]
        n167 = Enqueue Element(queue=w493, element=acquire_enum."Acquire") -> (queue out=w492:refnum<queue>)  [unwired: 2 in, 2 out]
        n168 = VISA Write(VISA resource name=w508, write buffer="c", error in (no error)=w509) -> (VISA resource name out=w481:refnum<visa-resource-name>, error out=w480:errorcluster)  [unwired: 1 out]
        n169 = call "send_mark_10_config.vi"("Number of Cycles"=w486, "VISA Refnum in"=w481, "error in (no error)"=w480, "Down Limit(mm)"=w485, "Up Limit(mm)"=w484, "Speed (mm/min)"=w487) -> ("error out"=w479:errorcluster, "VISA Refnum out"=w482:refnum<visa-resource-name>)  [unwired: 4 in]
      }
      frame "Open Mark-10 Setup" {
        n170 = call "mark_10_config_panel.vi"("Error In"=w546, "Mark-10 Settings"=w545) -> ("Error Out"=w551:errorcluster, "Mark-10 Settings 2"=w544:T2)  [unwired: 8 in]
        n171 = Unbundle By Name(w544) -> ("Speed (mm/min)"=w537:dbl, "Up Limit(mm)"=w548:dbl, "Down Limit(mm)"=w549:dbl, "Number of Cycles"=w550:i32)
        n172 = Get Queue Status(queue=w555) -> (queue out=w554:refnum<queue>, # elements in queue=w558:i32)  [unwired: 2 in, 6 out]
        n173 = call "visa_write.vi"("error in (no error)"=w551, "String"="c", "VISA Refnum in"=w547) -> ("error out"=w553:errorcluster, "VISA Refnum out"=w536:refnum<visa-resource-name>)  [unwired: 6 in]
        n174 = Equal To 0?(x=w558) -> (x = 0?=w557:bool)
        n175 = case shown="True" w557 {
          tunnel: w554 -> [w559 w562]
          tunnel: [w559 w561] -> w556
          frame False {
          }
          frame True {
            n176 = Enqueue Element(queue=w562, element=acquire_enum."Acquire") -> (queue out=w561:refnum<queue>)  [unwired: 2 in, 2 out]
          }
        }
        n177 = call "send_mark_10_config.vi"("Number of Cycles"=w550, "VISA Refnum in"=w536, "error in (no error)"=w553, "Down Limit(mm)"=w549, "Up Limit(mm)"=w548, "Speed (mm/min)"=w537) -> ("error out"=w542:errorcluster, "VISA Refnum out"=w543:refnum<visa-resource-name>)  [unwired: 4 in]
      }
      frame "Reset Cycle" {
        n178 = Get Queue Status(queue=w574) -> (queue out=w576:refnum<queue>, # elements in queue=w578:i32)  [unwired: 2 in, 6 out]
        n179 = Equal To 0?(x=w578) -> (x = 0?=w577:bool)
        n180 = case shown="True" w577 {
          tunnel: w576 -> [w579 w582]
          tunnel: [w579 w581] -> w575
          frame False {
          }
          frame True {
            n181 = Enqueue Element(queue=w582, element=acquire_enum."Acquire") -> (queue out=w581:refnum<queue>)  [unwired: 2 in, 2 out]
          }
        }
        n182 = call "visa_write.vi"("error in (no error)"=w571, "String"="t", "VISA Refnum in"=w572) -> ("error out"=w569:errorcluster, "VISA Refnum out"=w570:refnum<visa-resource-name>)  [unwired: 6 in]
      }
      frame "Connect to Mark-10" {
        w583 = u16 2 items=["None", "Last Bit", "TermChar", "Break"] ("Serial Settings:End Mode for Writes")
        w604 = TRUE
        w603 = u8 13 ("Termination Character")
        n183 = Unbundle By Name(T5 {"baud rate"=115200, "data bits"=8, "parity"=enum."None", "stop bits"=10, "flow control"=0, "IsConfigured"=FALSE} ("Serial Settings")) -> ("baud rate"=w606:u32, "data bits"=w607:u16, "parity"=w608:enum16{"None", "Odd", "Even", "Mark", "Space"}, "stop bits"=w609:u16, "flow control"=w610:u16)
        n184 = call-poly "VISA Configure Serial Port"("VISA resource name"=w594, "termination char\n(0xA = '\\n' = LF)"=w603, "Enable Termination\nChar (T)"=w604, "baud rate (9600)"=w606, "data bits (8)"=w607, "parity (0:none)"=w608, "stop bits (10: 1 bit)"=w609, "flow control (0:none)"=w610) -> ("VISA resource name out"=w611:refnum<visa-resource-name>, "error out"=w612:errorcluster)  [unwired: 6 in]
        n185 = property class="Instr"(reference=w611, error in=w612, "Serial Settings:End Mode for Writes"=w583, "Message Based Settings:Send End Enable"=w604, "Message Based Settings:Termination Character"=w603) -> (reference out=w615:refnum<visa-resource-name>, error out=w616:errorcluster)
        n186 = Enqueue Element(queue=w600, element=acquire_enum."Connect to NIDAQ") -> (queue out=w599:refnum<queue>)  [unwired: 2 in, 2 out]
        n187 = Unbundle By Name(w589) -> ("Speed (mm/min)"=w590:dbl, "Up Limit(mm)"=w591:dbl, "Down Limit(mm)"=w592:dbl, "Number of Cycles"=w593:i32)
        n188 = VISA Clear(VISA resource name=w615, error in (no error)=w616) -> (VISA resource name out=w613:refnum<visa-resource-name>, error out=w614:errorcluster)
        n189 = VISA Write(VISA resource name=w613, write buffer="i", error in (no error)=w614) -> (VISA resource name out=w587:refnum<visa-resource-name>, error out=w588:errorcluster)  [unwired: 1 out]
        n190 = call "send_mark_10_config.vi"("Number of Cycles"=w593, "VISA Refnum in"=w587, "error in (no error)"=w588, "Down Limit(mm)"=w592, "Up Limit(mm)"=w591, "Speed (mm/min)"=w590) -> ("error out"=w584:errorcluster, "VISA Refnum out"=w586:refnum<visa-resource-name>)  [unwired: 4 in]
      }
      frame "Connect to NIDAQ" {
        n191 = call <vilib>:"DAQmx Clear Task.vi"("task in"=w619) -> ()  [unwired: 14 in, 1 out]
        n192 = call "task_generator.vi"("rate"=w617) -> ("task out"=w630:refnum<k21>)  [unwired: 9 in, 1 out]
        n193 = call <vilib>:"DAQmx Start Task.vi"("task/channels in"=w630) -> ("task out"=w629:refnum<k21>)  [unwired: 13 in, 1 out]
        n194 = Enqueue Element(queue=w622, element=acquire_enum."New Log Path") -> (queue out=w621:refnum<queue>)  [unwired: 2 in, 2 out]
      }
      frame "Move to Target" {
        n195 = call "visa_write_after_read.vi"("error in (no error)"=w660, "String"="x", "VISA Refnum in"=w668) -> ("error out"=w646:errorcluster, "VISA Refnum out"=w645:refnum<visa-resource-name>, "Numeric"=w667:dbl)  [unwired: 5 in, 1 out]
        n196 = Flush Queue(queue=w655) -> (queue out=w654:refnum<queue>)  [unwired: 1 in, 2 out]
        n197 = Less?(x=w667, y="Target Distance") -> (x < y?=w666:bool)
        n198 = call "send_mark_10_config.vi"("Number of Cycles"=0, "VISA Refnum in"=w645, "error in (no error)"=w646, "Down Limit(mm)"=-500.0, "Up Limit(mm)"=500.0, "Speed (mm/min)"=1100.0) -> ("error out"=w634:errorcluster, "VISA Refnum out"=w636:refnum<visa-resource-name>)  [unwired: 4 in]
        n199 = case shown="False" w666 {
          tunnel: ["d" "u"] -> w632
          frame False {
          }
          frame True {
          }
        }
        n200 = call "visa_write.vi"("error in (no error)"=w634, "String"=w632, "VISA Refnum in"=w636) -> ("error out"=w633:errorcluster, "VISA Refnum out"=w635:refnum<visa-resource-name>)  [unwired: 6 in]
        n201 = while {
          tunnel: w635 -> [w691]
          tunnel: "Target Distance" -> [w682]
          tunnel: [w684] -> w659
          tunnel: [w683] -> w658
          tunnel: w654 -> [w679]
          tunnel: [w678] -> w652
          tunnel: w633 -> [w674]
          stop <- w676 stop-if-true
          n202 = call "visa_write_after_read.vi"("error in (no error)"=w674, "String"="x", "VISA Refnum in"=w691) -> ("error out"=w685:errorcluster, "VISA Refnum out"=w686:refnum<visa-resource-name>, "Numeric"=w690:dbl)  [unwired: 5 in, 1 out]
          n203 = Subtract(x=w690, y=w682) -> (x-y=w689:dbl)
          n204 = Absolute Value(x=w689) -> (abs(x)=w672:dbl)
          n205 = Greater?(x=10.0, y=w672) -> (0:w687:bool)
          n206 = Less?(x=w672, y=0.04) -> (x < y?=w675:bool)
          n207 = Get Queue Status(queue=w679) -> (queue out=w678:refnum<queue>, # elements in queue=w681:i32)  [unwired: 2 in, 6 out]
          n208 = case shown="True" w687 {
            tunnel: w686 -> [w694 w698]
            tunnel: w685 -> [w693 w697]
            tunnel: [w694 w696] -> w684
            tunnel: [w693 w695] -> w683
            frame False {
            }
            frame True {
              n209 = call "speed_limit_setup.vi"("Speed"=100.0) -> ("String out 3"=w700:string)  [unwired: 8 in, 2 out]
              n210 = call "visa_write.vi"("error in (no error)"=w697, "String"=w700, "VISA Refnum in"=w698) -> ("error out"=w695:errorcluster, "VISA Refnum out"=w696:refnum<visa-resource-name>)  [unwired: 6 in]
            }
          }
          n211 = Not Equal?(x=w681, y=0) -> (x != y?=w677:bool)
          n212 = Or(x=w677, y=w675) -> (x .or. y?=w676:bool)
        }
        n213 = Unbundle By Name(w656) -> ("Speed (mm/min)"=w640:dbl, "Up Limit(mm)"=w639:dbl, "Down Limit(mm)"=w638:dbl, "Number of Cycles"=w637:i32)
        n214 = call "visa_write.vi"("error in (no error)"=w658, "String"="s", "VISA Refnum in"=w659) -> ("error out"=w642:errorcluster, "VISA Refnum out"=w644:refnum<visa-resource-name>)  [unwired: 6 in]
        n215 = Enqueue Element(queue=w652, element=acquire_enum."Acquire") -> (queue out=w651:refnum<queue>)  [unwired: 2 in, 2 out]
        n216 = call "send_mark_10_config.vi"("Number of Cycles"=w637, "VISA Refnum in"=w644, "error in (no error)"=w642, "Down Limit(mm)"=w638, "Up Limit(mm)"=w639, "Speed (mm/min)"=w640) -> ("error out"=w641:errorcluster, "VISA Refnum out"=w643:refnum<visa-resource-name>)  [unwired: 4 in]
      }
    }
  }
  n217 = Flush Queue(queue=w25) -> (queue out=w36:refnum<queue>, error out=w34:errorcluster)  [unwired: 1 in, 1 out]
  n218 = Release Queue(queue=w36, error in (no error)=w34) -> ()  [unwired: 1 in, 3 out]
  n219 = Close File(refnum=w32) -> ()  [unwired: 1 in, 2 out]
  n220 = call <vilib>:"DAQmx Clear Task.vi"("task in"=w33) -> ()  [unwired: 14 in, 1 out]
  n221 = VISA Close(VISA resource name=w26) -> ()  [unwired: 1 in, 1 out]
  n222 = Flush Queue(queue=w24) -> (queue out=w23:refnum<queue>)  [unwired: 1 in, 2 out]
  n223 = Release Queue(queue=w23) -> ()  [unwired: 2 in, 3 out]
